vi "jrg_eod_file_position.vi"(8 "error in (no error)":errorcluster, 10 "operation":T1(ring)=enum."open or create", 11 "Refnum in":refnum<file>) -> (0 "error out":errorcluster, 3 "Refnum out":refnum<file>)   [LabVIEW 2014]
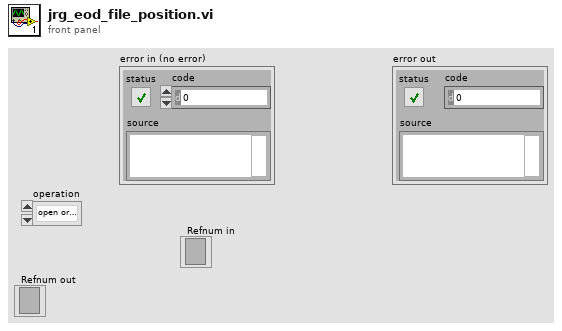
[diagram p1: front panel]
types:
  T1 = enum16{"open", "replace", "create", "open or create", "replace or create", "replace or create with confirmation"}
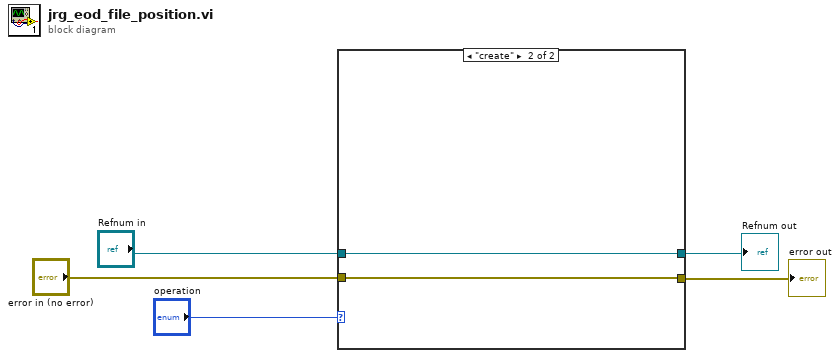
[diagram p0: block diagram]
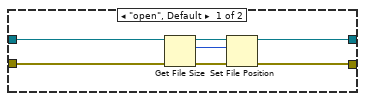
[diagram p2: hidden frame]
diagram:
  n1 = case shown="\"create\"" "operation" {
    tunnel: "Refnum in" -> [w7 w14]
    tunnel: "error in (no error)" -> [w8 w13]
    tunnel: [w6 w14] -> w2
    tunnel: [w9 w13] -> w4
    frame "open", Default {
      n2 = Get File Size(file=w7, error in=w8) -> (refnum out=w12:refnum<file>, size (in bytes)=w10:i64, 0:w11:errorcluster)
      n3 = Set File Position(offset (in bytes) (0)=w10, refnum=w12, error in=w11) -> (refnum out=w6:refnum<file>, error out=w9:errorcluster)  [unwired: 1 in]
    }
    frame "create" {
    }
  }
  "error out" <- w4
  "Refnum out" <- w2
